vi "Characteristic_Value_C_FGV.vi"(7 "Command":enum16{"SET", "GET"}(ring), 8 "error in (no error)":errorcluster, 11 "Characteristic_Value_C_IN":dbl) -> (0 "error out":errorcluster, 3 "Characteristic_Value_C_OUT":dbl)   [LabVIEW 2017]
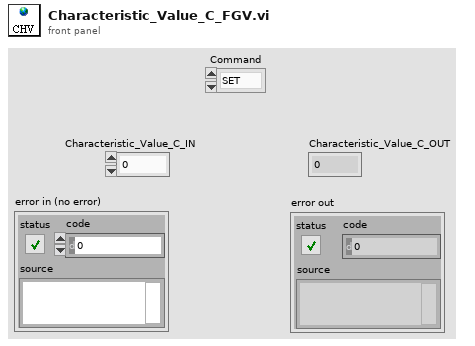
[diagram p1: front panel]
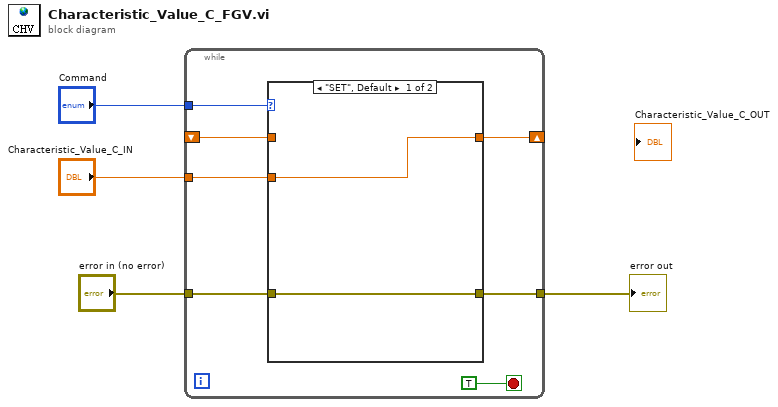
[diagram p0: block diagram]
diagram:
  n1 = while {
    shift-right: [w9] -> _
    shift-left: _ -> [w7]
    tunnel: "Command" -> [w10]
    tunnel: "Characteristic_Value_C_IN" -> [w8]
    tunnel: [w6] -> w2
    tunnel: "error in (no error)" -> [w5]
    stop <- TRUE stop-if-true
    n2 = case shown="\"SET\", Default" w10 {
      tunnel: [w13 w15] -> w9
      tunnel: w8 -> [w13 _]
      tunnel: w7 -> [_ w15]
      tunnel: [w12 w14] -> w6
      tunnel: w5 -> [w12 w14]
      frame "SET", Default {
      }
      frame "GET" {
      }
    }
  }
  "error out" <- w2
